vi "GDSAPI_Example_CreateMethods2.vi"() -> ()   [LabVIEW 2012]
uses:
  <resource>/Framework/Providers/Open_GDS/API/GDSAPI_SubVIs/GDSAPI_ClassProviderType.ctl
  <resource>/Framework/Providers/Open_GDS/API/GDSAPI_CreateClassType.ctl
  <resource>/Framework/Providers/Open_GDS/API/GDSAPI_SubVIs/GDSAPI_ClassTemplateType.ctl
  <resource>/Framework/Providers/Open_GDS/ClassProviders/Common/CommonVIs/CommonVIs_AttributeType.ctl
  <resource>/Framework/Providers/Open_GDS/ClassProviders/Common/CommonVIs/CommonVIs_AttributeDataType.ctl
  <resource>/Framework/Providers/Open_GDS/ClassProviders/Common/String/GDSString_AccessScopeModifierType.ctl
  <resource>/Framework/Providers/Open_GDS/ClassProviders/Common/String/GDSString_MethodDescriptionType.ctl
  <resource>/Framework/Providers/Open_GDS/ClassProviders/Common/String/GDSString_ModifierType.ctl
  <resource>/Framework/Providers/Open_GDS/ClassProviders/Common/CommonVIs/CommonVIs_PropertyType.ctl
panel:
  out "error out":errorcluster
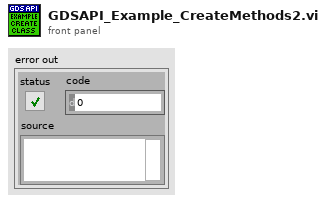
[diagram p1: front panel]
types:
  T1 = typedef "GDSString_MethodDescriptionType.ctl" = cluster{"ReturnType":T2, "MethodName":string, "AccessScope":T4, "Modifiers":T5[], "MethodDocumentation":string, "MethodContent":string, "MethodArguments":T2[], "GetProperty":T6, "SetProperty":T6}
  T2 = typedef "CommonVIs_AttributeType.ctl" = cluster{"Name":string, "DataType":T3, "ArrayDim":i32, "CtrlPath":path, "DataTypeString":string, "AccessScope":T4, "InitialData":variant}
  T3 = typedef "CommonVIs_AttributeDataType.ctl" = enum16{"UINT8", "INT8", "UINT16", "INT16", "UINT32", "INT32", "UINT64", "INT64", "SGL", "DBL", "EXT", "CSG", "CDB", "CXT", "TimeStamp", "STRING", "PATH", "BOOL", "ENUM", "RefNum", "VIRefNum", "LabVIEW Class", "Cluster", "Variant", "TypeDef", "Waveform", "LabVIEW Object", "Other", "void"}
  T4 = typedef "GDSString_AccessScopeModifierType.ctl" = enum16{"public", "private", "protected", "internal"}
  T5 = typedef "GDSString_ModifierType.ctl" = enum16{"abstract", "static", "final", "synchronized", "strictfp", "async", "const", "event", "extern", "new", "native ", "override", "partial", "readonly", "sealed", "unsafe", "virtual", "volatile"}
  T6 = typedef "CommonVIs_PropertyType.ctl" = cluster{"Active":bool, "AccessScope":T4, "Code":string}
  T7 = typedef "GDSAPI_CreateClassType.ctl" = cluster{"ClassProvider":T8, "NewClassFolder":path, "ParentLvClassFilePath":path, "ClassName":string, "ClassDescription":string, "ClassTemplate":T9}
  T8 = typedef "GDSAPI_ClassProviderType.ctl" = enum16{"LabVIEW Native(By value)", "GOOP-3(By reference)", "GOOP-4(By reference)"}
  T9 = typedef "GDSAPI_ClassTemplateType.ctl" = enum16{"Standard", "Singleton", "Interface(By Aggregation)", "Interface(By VI Server)"}
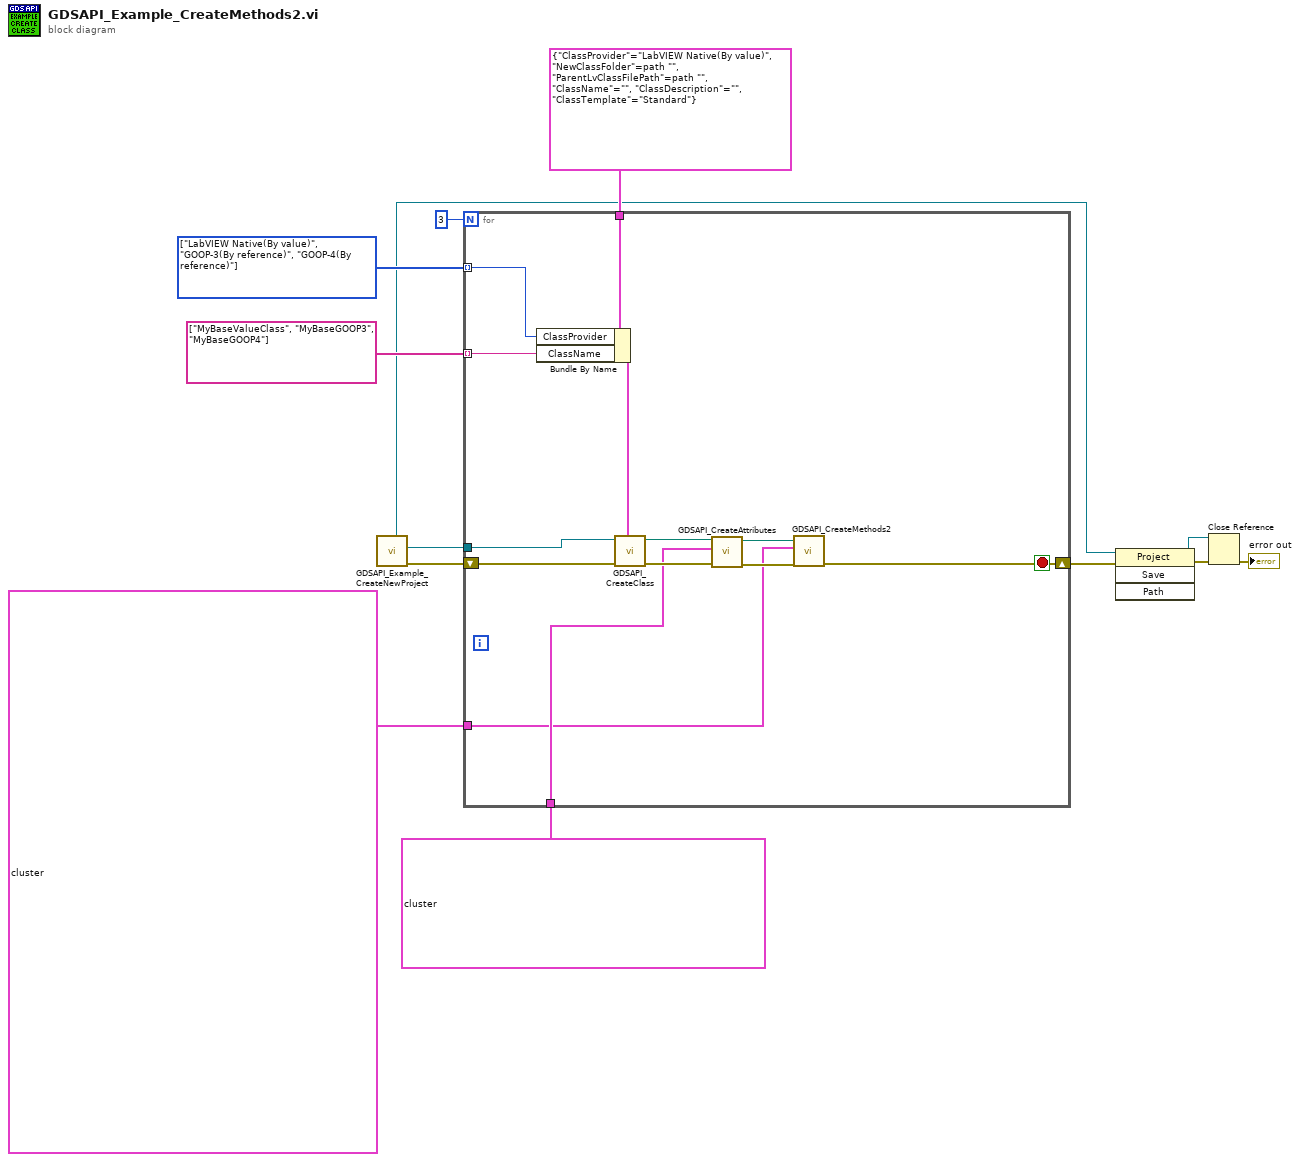
[diagram p0: block diagram]
diagram:
  w7 = T8[] [enum."LabVIEW Native(By value)", enum."GOOP-3(By reference)", enum."GOOP-4(By reference)"] items=["LabVIEW Native(By value)", "GOOP-3(By reference)", "GOOP-4(By reference)"]
  n1 = call <resource>:"GDSAPI_Example_CreateNewProject.vi"() -> ("error out"=w13:errorcluster, "ProjectItem out"=w12:refnum<vi>, "ProjectRefOut"=w6:refnum<vi>)  [unwired: 8 in, 1 out]
  n2 = for {
    N: 3 -> [_]
    tunnel: w12 -> [w26]
    tunnel: T7 {"ClassProvider"=enum."LabVIEW Native(By value)", "NewClassFolder"=path "", "ParentLvClassFilePath"=path "", "ClassName"="", "ClassDescription"="", "ClassTemplate"=enum."Standard"} ("CreateClassType") -> [w25]
    tunnel: string[] ["MyBaseValueClass", "MyBaseGOOP3", "MyBaseGOOP4"] -> [w23] mode=indexing
    tunnel: w7 -> [w22] mode=indexing
    shift-right: [w14] -> w3
    shift-left: w13 -> [w21]
    tunnel: T2[] [{"Name"="EmailsToSendTo", "DataType"=enum."STRING", "ArrayDim"=1, "CtrlPath"=path "", "DataTypeString"="", "AccessScope"=enum."public", "InitialData"=variant}, {"Name"="SmtpServer", "DataType"=enum."STRING", "ArrayDim"=0, "CtrlPath"=path "", "DataTypeString"="", "AccessScope"=enum."public", "InitialData"=variant}, {"Name"="SmtpPort", "DataType"=enum."INT16", "ArrayDim"=0, "CtrlPath"=path "", "DataTypeString"="", "AccessScope"=enum."public", "InitialData"=variant}, {"Name"="EmailToSendFrom", "DataType"=enum."STRING", "ArrayDim"=0, "CtrlPath"=path "", "DataTypeString"="", "AccessScope"=enum."public", "InitialData"=variant}, {"Name"="PasswordToSendFrom", "DataType"=enum."STRING", "ArrayDim"=0, "CtrlPath"=path "", "DataTypeString"="", "AccessScope"=enum."public", "InitialData"=variant}] ("Attributes") -> [w16]
    tunnel: T1[] [{"ReturnType"={"Name"="", "DataType"=enum."STRING", "ArrayDim"=1, "CtrlPath"=path "", "DataTypeString"="List<String>", "AccessScope"=enum."public", "InitialData"=variant(string "")}, "MethodName"="EmailsToSendTo", "AccessScope"=enum."public", "Modifiers"=[], "MethodDocumentation"="", "MethodContent"="public List<String> EmailsToSendTo { get; set; }", "MethodArguments"=[], "GetProperty"={"Active"=TRUE, "AccessScope"=enum."public", "Code"=""}, "SetProperty"={"Active"=TRUE, "AccessScope"=enum."public", "Code"=""}}, {"ReturnType"={"Name"="", "DataType"=enum."STRING", "ArrayDim"=0, "CtrlPath"=path "", "DataTypeString"="String", "AccessScope"=enum."public", "InitialData"=variant(string "")}, "MethodName"="SmtpServer", "AccessScope"=enum."public", "Modifiers"=[], "MethodDocumentation"="", "MethodContent"="public String SmtpServer { get; set; }", "MethodArguments"=[], "GetProperty"={"Active"=TRUE, "AccessScope"=enum."public", "Code"=""}, "SetProperty"={"Active"=TRUE, "AccessScope"=enum."public", "Code"=""}}, {"ReturnType"={"Name"="", "DataType"=enum."INT16", "ArrayDim"=0, "CtrlPath"=path "", "DataTypeString"="short", "AccessScope"=enum."public", "InitialData"=variant(string "")}, "MethodName"="SmtpPort", "AccessScope"=enum."public", "Modifiers"=[], "MethodDocumentation"="", "MethodContent"="public short SmtpPort { get; set; }", "MethodArguments"=[], "GetProperty"={"Active"=TRUE, "AccessScope"=enum."public", "Code"=""}, "SetProperty"={"Active"=TRUE, "AccessScope"=enum."public", "Code"=""}}, {"ReturnType"={"Name"="", "DataType"=enum."STRING", "ArrayDim"=0, "CtrlPath"=path "", "DataTypeString"="String", "AccessScope"=enum."public", "InitialData"=variant(string "")}, "MethodName"="EmailToSendFrom", "AccessScope"=enum."public", "Modifiers"=[], "MethodDocumentation"="", "MethodContent"="public String EmailToSendFrom { get; set; }", "MethodArguments"=[], "GetProperty"={"Active"=TRUE, "AccessScope"=enum."public", "Code"=""}, "SetProperty"={"Active"=TRUE, "AccessScope"=enum."public", "Code"=""}}, {"ReturnType"={"Name"="", "DataType"=enum."STRING", "ArrayDim"=0, "CtrlPath"=path "", "DataTypeString"="String", "AccessScope"=enum."public", "InitialData"=variant(string "")}, "MethodName"="PasswordToSendFrom", "AccessScope"=enum."public", "Modifiers"=[], "MethodDocumentation"="", "MethodContent"="public String PasswordToSendFrom { get; set; }", "MethodArguments"=[], "GetProperty"={"Active"=TRUE, "AccessScope"=enum."public", "Code"=""}, "SetProperty"={"Active"=TRUE, "AccessScope"=enum."public", "Code"=""}}] ("Methods") -> [w15]
    stop <- w14 stop-if-true
    n3 = Bundle By Name(cluster=w25, "ClassProvider"=w22, "ClassName"=w23) -> (w24:T7)
    n4 = call <resource>:"GDSAPI_CreateClass.vi"("error in (no error)"=w21, "CreateClassType"=w24, "ProjectItem"=w26) -> ("error out"=w20:errorcluster, "LvClassFileOut"=w18:path)  [unwired: 6 in, 1 out]
    n5 = call <resource>:"GDSAPI_CreateAttributes.vi"("error in (no error)"=w20, "Attributes"=w16, "ClassPath(*.lvclass)"=w18) -> ("error out"=w19:errorcluster, "ClassPathOut(*.lvclass)"=w17:path)  [unwired: 7 in]
    n6 = call <resource>:"GDSAPI_CreateMethods2.vi"("error in (no error)"=w19, "Methods"=w15, "ClassPath(*.lvclass)"=w17) -> ("error out"=w14:errorcluster)  [unwired: 8 in]
  }
  n7 = invoke class="Project" method="Save"(reference=w6, error in=w3) -> (reference out=w10:refnum<vi>, error out=w11:errorcluster)  [unwired: 2 in, 2 out]
  n8 = Close Reference(reference=w10, error in (no error)=w11) -> (error out=→"error out":errorcluster)
